vi "ex4_visual output.vi"() -> ()   [LabVIEW 2018]
panel:
  out "Waveform Graph":dbl[](graph)
  out "Waveform Chart":dbl(graph)
  out "Numeric":dbl
  in  "stop":bool
  in  "Knob":dbl(knob) scale=0.2..200.0
  out "Thermometer":dbl(slide) scale=0.0..100.0
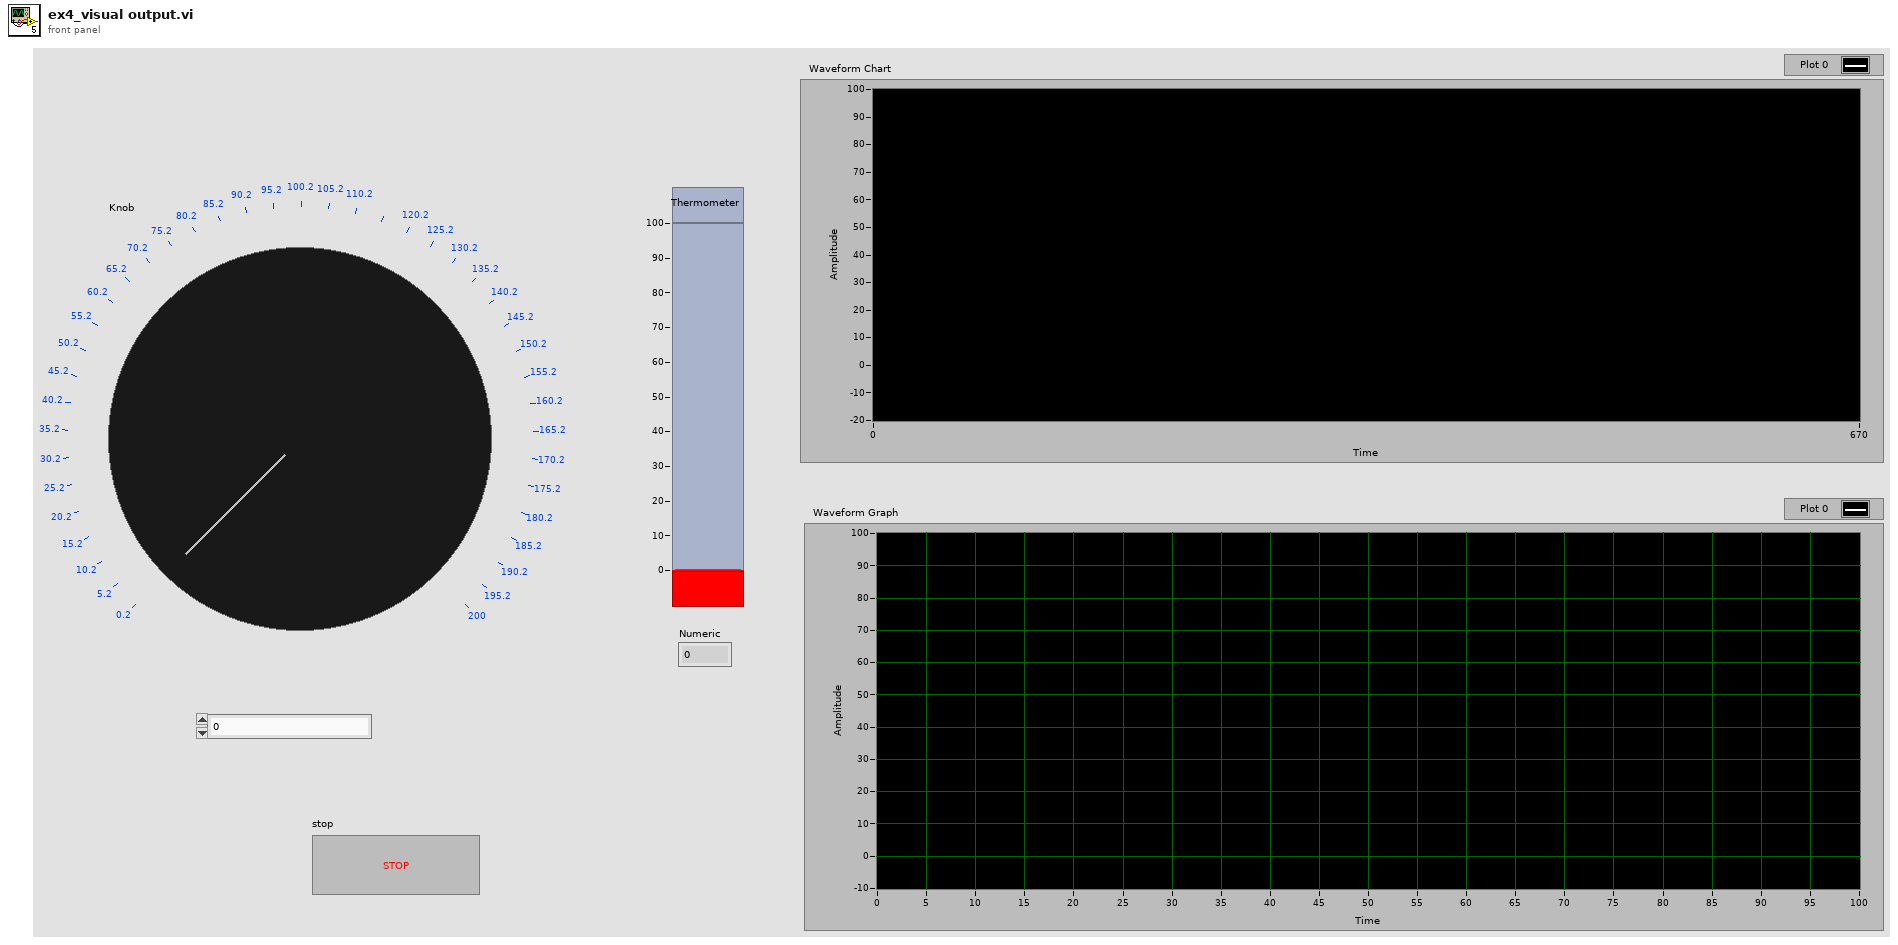
[diagram p1: front panel]
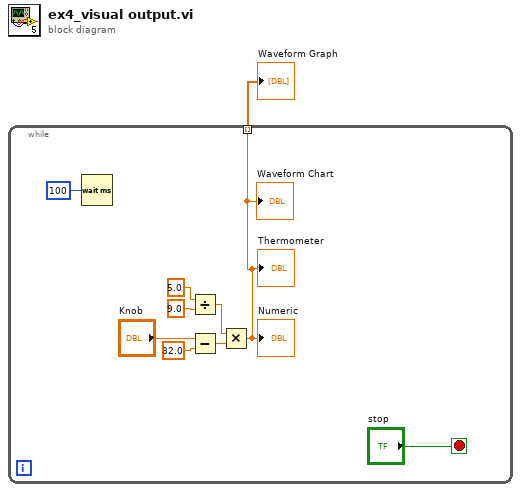
[diagram p0: block diagram]
diagram:
  n1 = while {
    tunnel: [w2] -> w1 mode=indexing
    stop <- "stop" stop-if-true
    n2 = Wait (ms)(milliseconds to wait=100) -> ()  [unwired: 1 out]
    n3 = Divide(x=5.0, y=9.0) -> (x/y=w5:dbl)
    n4 = Subtract(x="Knob", y=32.0) -> (x-y=w4:dbl)
    n5 = Multiply(x=w5, y=w4) -> (x*y=w2:dbl)
    "Thermometer" <- w2
    "Numeric" <- w2
    "Waveform Chart" <- w2
  }
  "Waveform Graph" <- w1
